vi "UUT select.vi"(8 "error constant":errorcluster, 11 "UUT":u16(ring)=3 items=["BLDC 60A"=1, "BLDC 30A"=2, "Warrior 60A"=3]) -> (0 "error constant 2":errorcluster, 2 "UUT Out":string, 3 "UUT Out":u16(ring)=3 items=["BLDC  60A  P/N: 1"=1, "BLDC  30A  P/N: 2"=2, "Warrior 60A P/N: 3"=3, "Condenser Merkava P/N: 4"=4, "Condenser India P/N: 4"=5])   [LabVIEW 2017]
panel:
  in  "Next Button":bool
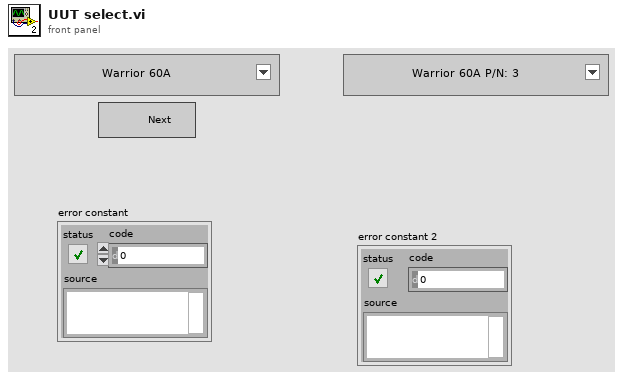
[diagram p1: front panel]
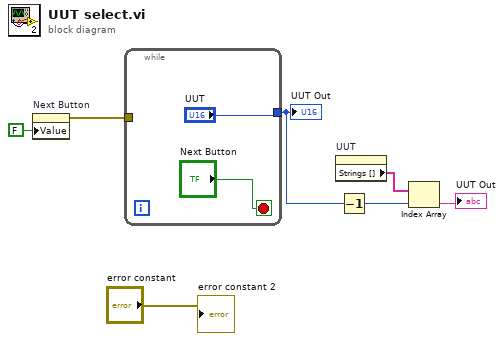
[diagram p0: block diagram]
diagram:
  n1 = property on="Next Button" class="Bool (strict)"("Value"=FALSE ("Next Button")) -> (error out=w5:errorcluster)  [unwired: 2 in, 1 out]
  n2 = while {
    tunnel: ["UUT"] -> w3
    tunnel: w5 -> [_]
    stop <- "Next Button" stop-if-true
  }
  "UUT Out" <- w3
  n3 = property on="UUT" class="Ring (strict)"() -> ("Strings []"=w4:string[])  [unwired: 2 in, 2 out]
  n4 = Decrement(x=w3) -> (x-1=w1:u16)
  n5 = Index Array(array=w4, index=w1) -> (element=→"UUT Out":string)
  "error constant 2" <- "error constant"
